vi "(Depricated) Write Sample Push.Sample mBar.vi"(10 "Sample mBar":dbl, 11 "cRIO-CO2 in":refnum<class "cRIO-CO2.lvclass">) -> (3 "cRIO-CO2 out":refnum<class "cRIO-CO2.lvclass">)   [LabVIEW 2015]
uses:
  cRIO-CO2.lvclass
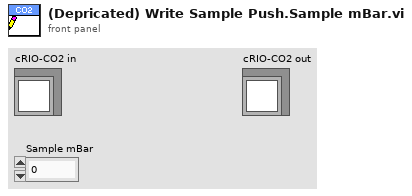
[diagram p1: front panel]
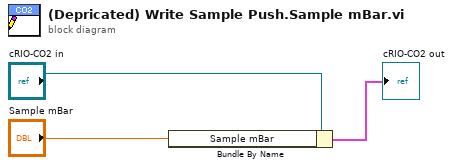
[diagram p0: block diagram]
diagram:
  n1 = Bundle By Name(cluster="cRIO-CO2 in", "Sample mBar"="Sample mBar") -> (→"cRIO-CO2 out":cluster{})
